vi "HelpBrowser.vi"() -> ()   [LabVIEW 2011]
uses:
  <vilib>/event_ctls.llb/eventvkey.ctl
panel:
  in  "Tab Control":T1(tab)
  in  "WebBrowser":refnum<k7>(container)
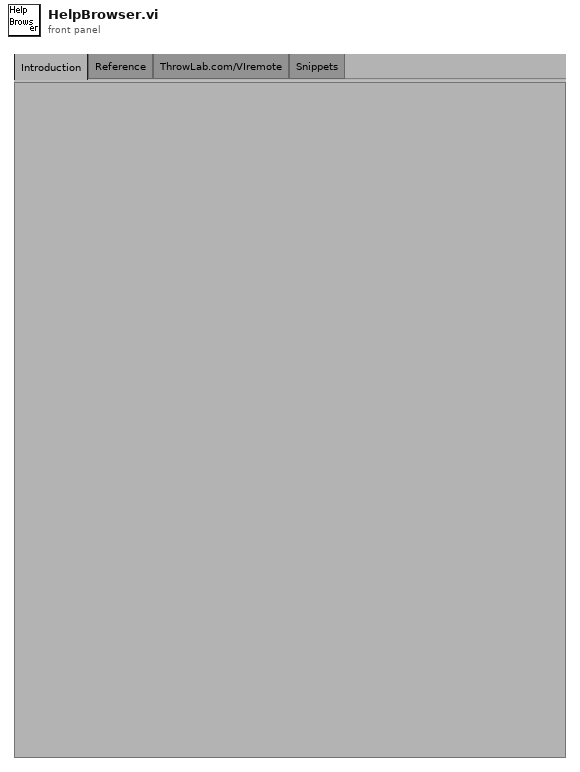
[diagram p1: front panel]
types:
  T1 = enum32{"Introduction", "Reference", "ThrowLab.com/VIremote", "Snippets"}
  T2 = typedef "eventvkey.ctl" = enum16{"ASCII", "Enter", "Return", "Shift", "Ctrl", "Alt", "Cmd", "Opt", "Caps", "NumLock", "Clear", "Break", "Up", "Down", "Left", "Right", "Insert", "Delete", "Home", "End", "PageUp", "PageDown", "Escape", "Help", "Pause", "ScrollLock", "F1", "F2", "F3", "F4", "F5", "F6", "F7", "F8", "F9", "F10", "F11", "F12", "F13", "F14", "F15", "F16", "F17", "F18", "F19", "F20", "F21", "F22", "F23", "F24", "Play", "VolumeUp", "VolumeDown", "Mute", "Two Byte Char"}
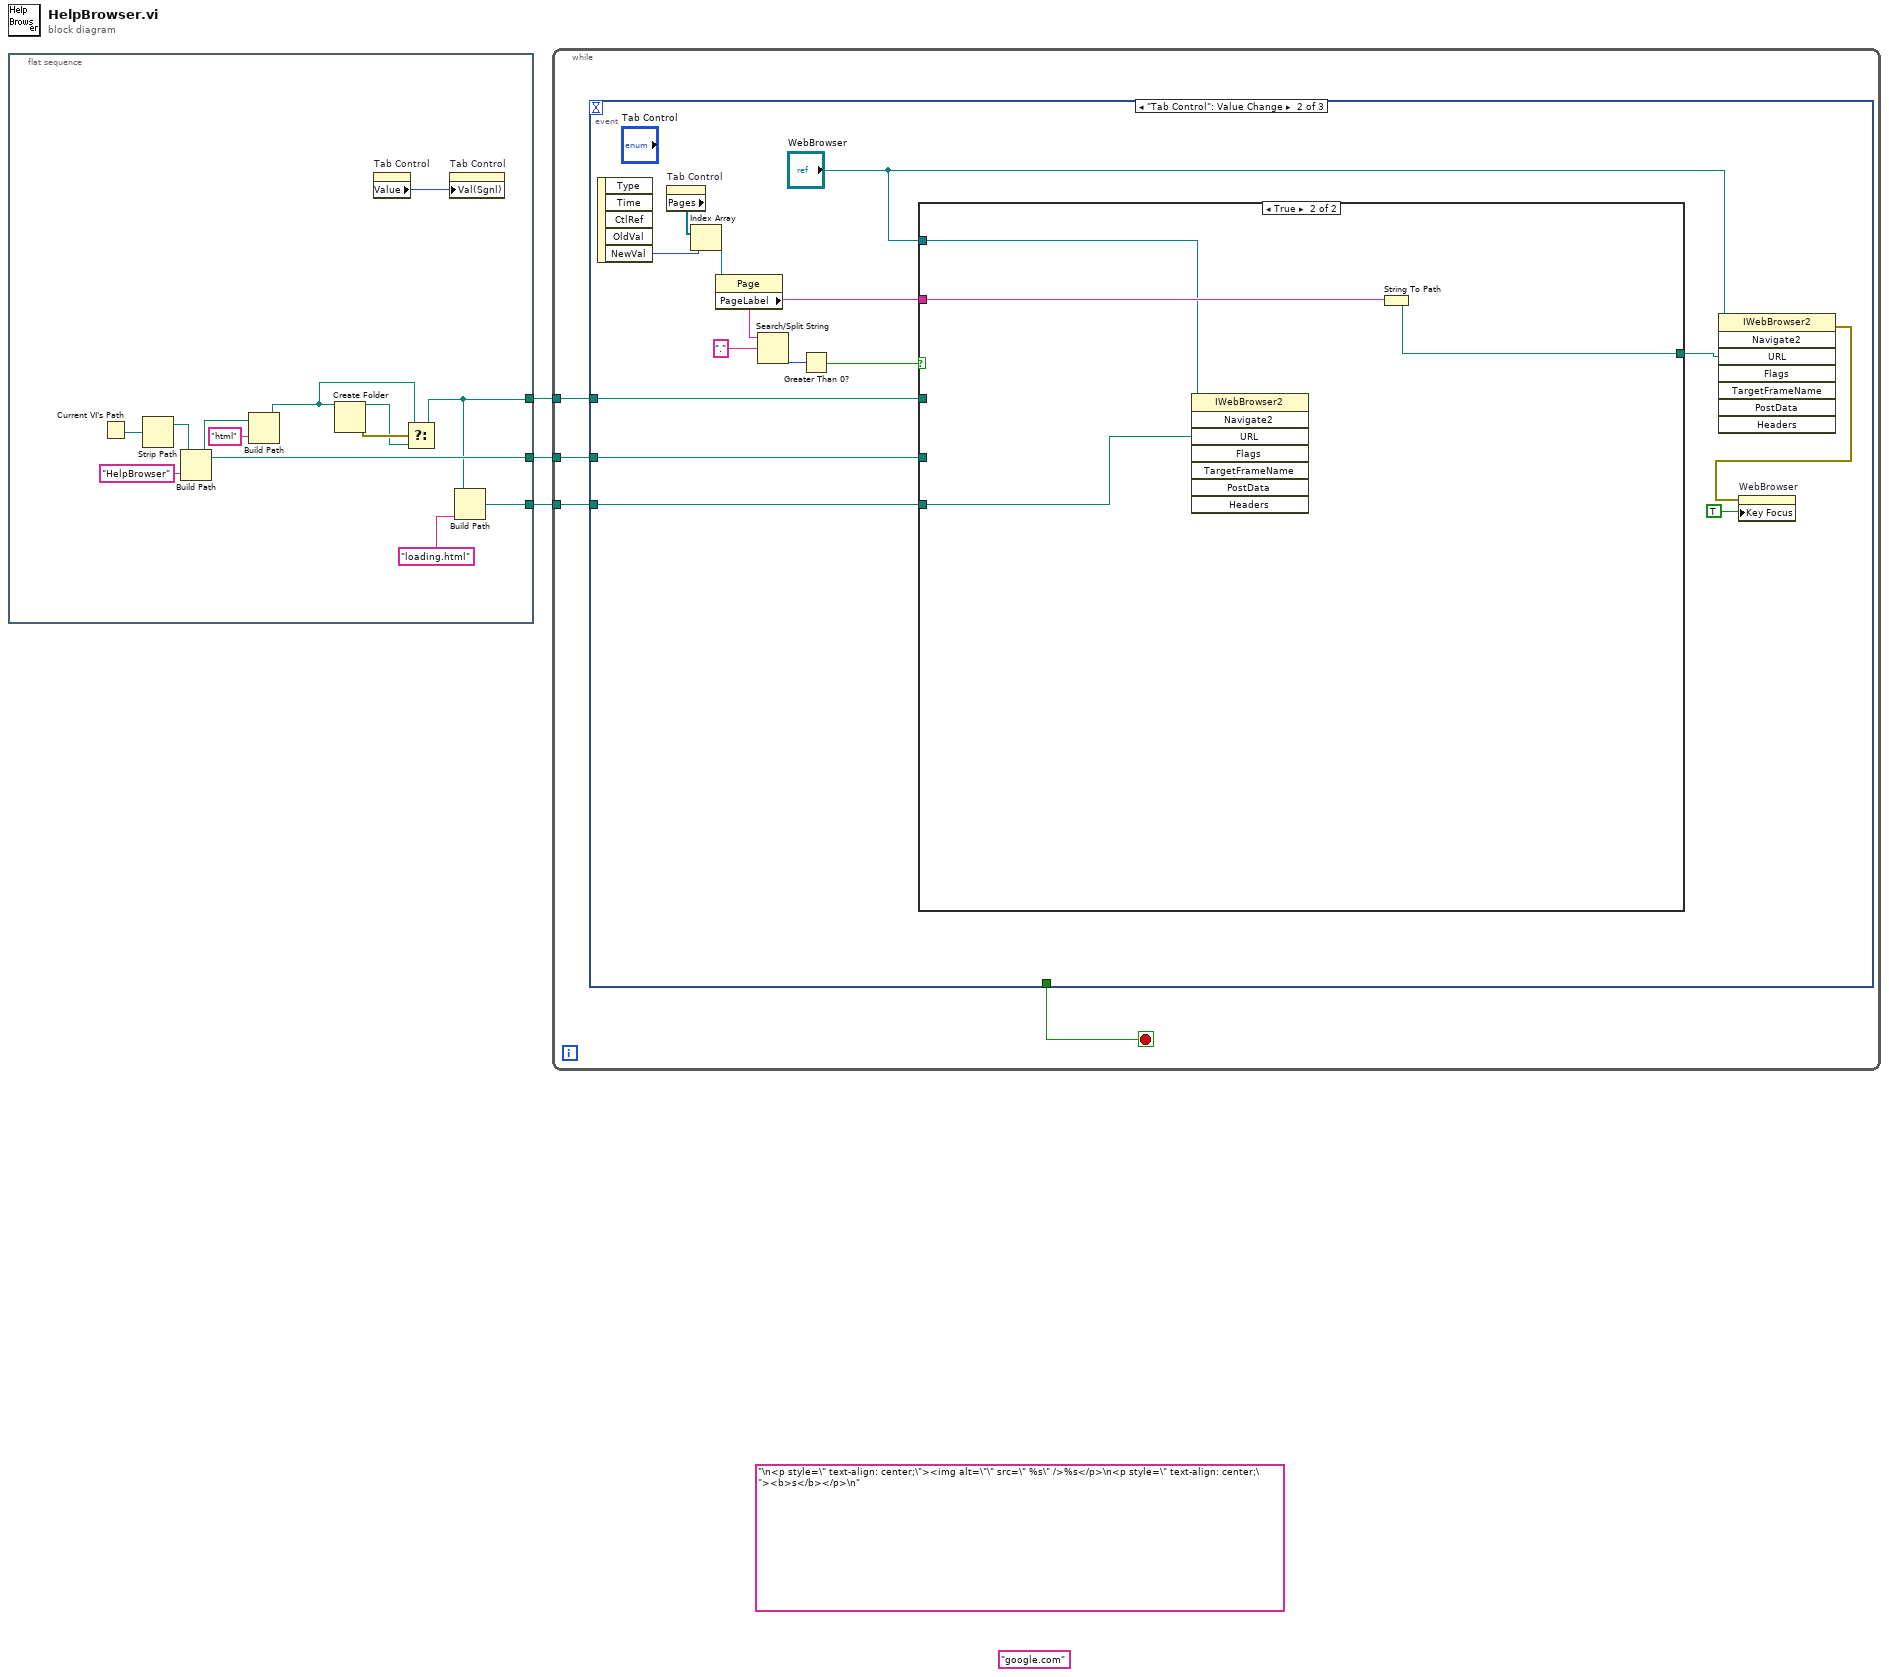
[diagram p0: block diagram]
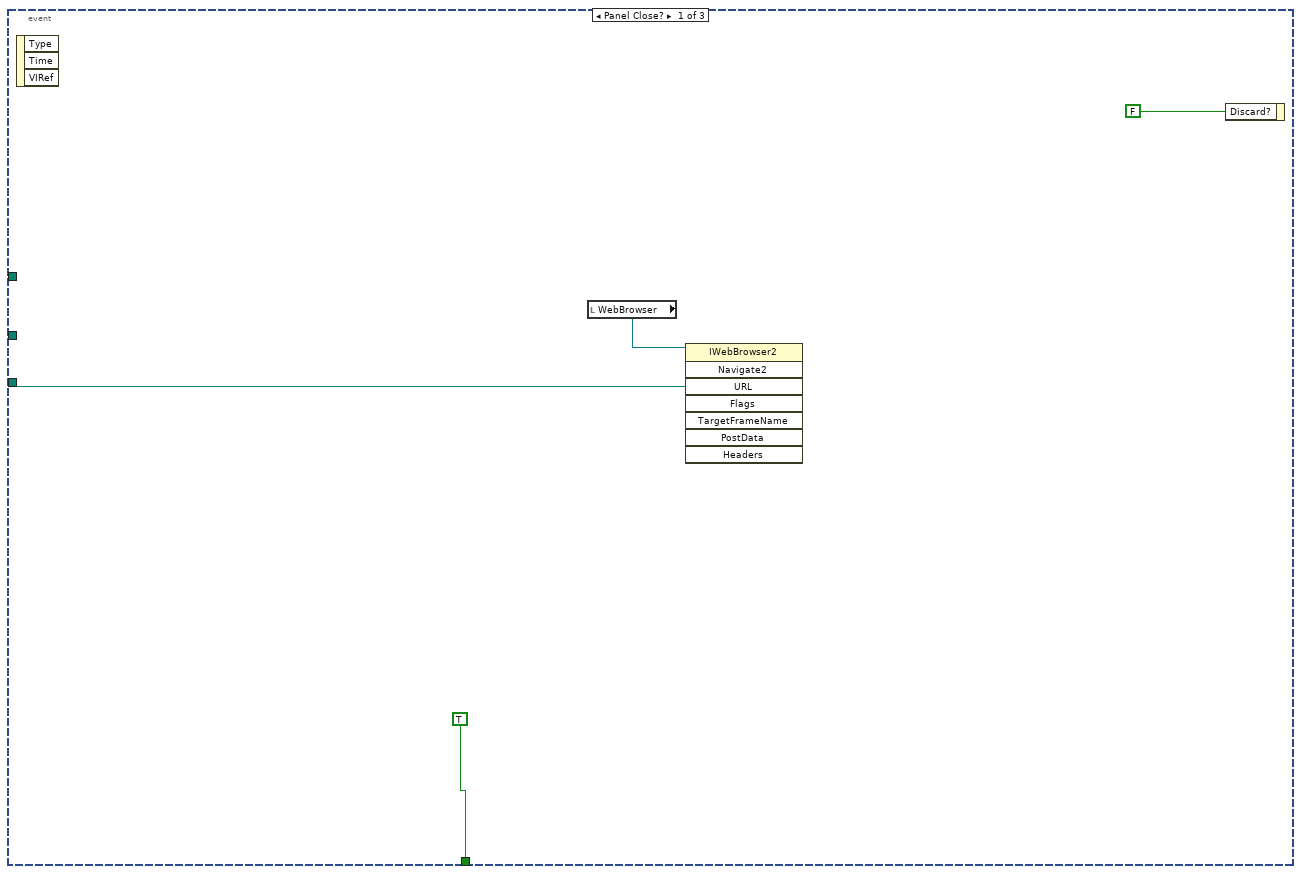
[diagram p2: hidden frame]
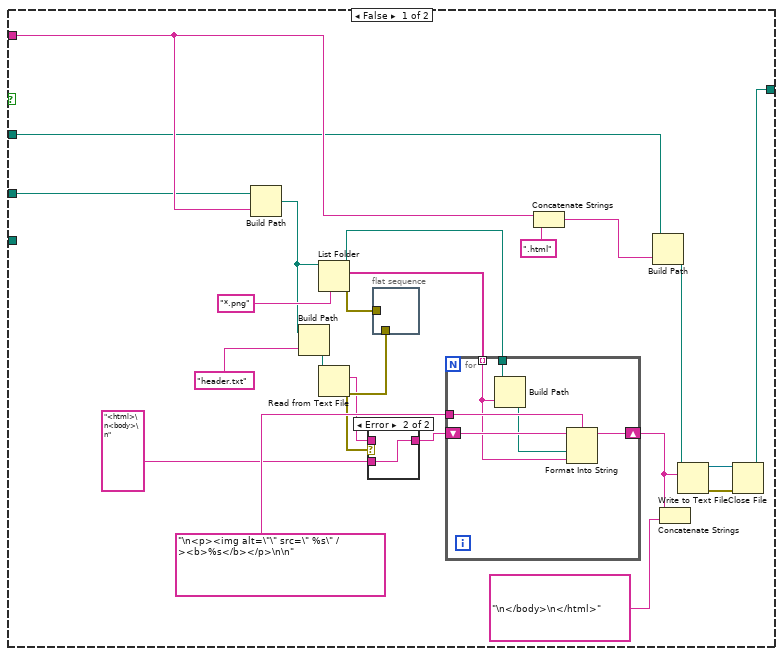
[diagram p3: hidden frame]
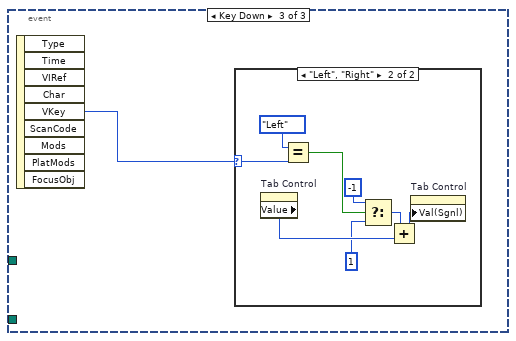
[diagram p5: hidden frame]
diagram:
  (unwired) "\n<p style=\" text-align: center;\"><img alt=\"\" src=\" %s\" />%s</p>\n<p style=\" text-align: center;\"><b>s</b></p>\n" ("name or relative path")
  (unwired) "google.com" ("URL")
  n1 = flat-sequence {
    tunnel: [w7] -> w3
    tunnel: [w5] -> w2
    tunnel: [w4] -> w1
    frame #0 {
      n2 = Current VI's Path() -> (path=w10:path)
      n3 = Strip Path(path=w10) -> (stripped path=w9:path)  [unwired: 1 out]
      n4 = Build Path(base path=w9, name or relative path="HelpBrowser") -> (appended path=w7:path)
      n5 = Build Path(base path=w7, name or relative path="html") -> (appended path=w14:path)
      n6 = Create Folder(path (use dialog)=w14) -> (created path=w12:path, error out=w13:errorcluster)  [unwired: 1 in, 2 out]
      n7 = property on="Tab Control" class="TabCtl (strict)"() -> ("Value"=w15:T1)  [unwired: 2 in, 2 out]
      n8 = Select(t=w14, s=w13, f=w12) -> (s? t:f=w5:path)
      n9 = property on="Tab Control" class="TabCtl (strict)"("Val(Sgnl)"=w15) -> ()  [unwired: 2 in, 2 out]
      n10 = Build Path(base path=w5, name or relative path="loading.html") -> (appended path=w4:path)
    }
  }
  n11 = while {
    tunnel: w2 -> [w18]
    tunnel: w3 -> [w17]
    tunnel: w1 -> [w16]
    stop <- w19 stop-if-true
    n12 = event shown="[1] \"Tab Control\": Value Change" {
      selector: _ -> [_ _ _]
      dyn-events: _ -> [_ _ _]
      timeout: _ -> [_ _ _]
      tunnel: [TRUE ("Discard?") _ _] -> w19
      tunnel: w18 -> [_ w27 _]
      tunnel: w17 -> [_ w26 _]
      tunnel: w16 -> [w21 w25 _]
      event Panel Close? {
        n13 = event-data() -> ()  [unwired: 4 out]
        n14 = local read "WebBrowser"() -> (w22:refnum<k7>)
        n15 = invoke class="IWebBrowser2" method="Navigate2"(reference=w22, "URL"=w21) -> ()  [unwired: 6 in, 8 out]
        n16 = event-data("Discard?"=FALSE) -> ()  [unwired: 1 in, 1 out]
      }
      event "Tab Control": Value Change {
        n17 = event-data() -> ("NewVal"=w37:T1)  [unwired: 5 out]
        n18 = property on="Tab Control" class="TabCtl (strict)"() -> ("Pages"=w36:refnum<vi>[])  [unwired: 2 in, 2 out]
        n19 = Index Array(array=w36, index=w37) -> (element=w35:refnum<vi>)
        n20 = property class="Page"(reference=w35) -> ("PageLabel"=w33:string)  [unwired: 1 in, 2 out]
        n21 = Search/Split String(string=w33, search string/char (-)=".") -> (offset of match=w31:i32)  [unwired: 3 out]
        n22 = Greater Than 0?(x=w31) -> (x > 0?=w30:bool)
        n23 = case shown="True" w30 {
          tunnel: [w57 w71] -> w34
          tunnel: w33 -> [w40 w72]
          tunnel: w26 -> [w39 _]
          tunnel: w27 -> [w38 _]
          tunnel: "WebBrowser" -> [_ w70]
          tunnel: w25 -> [_ w69]
          frame False {
            n24 = Build Path(base path=w39, name or relative path=w40) -> (appended path=w47:path)
            n25 = Build Path(base path=w47, name or relative path="header.txt" ("pattern")) -> (appended path=w48:path)
            n26 = List Folder(path=w47, pattern="*.png") -> (path out=w58:path, filenames=w53:string[], error out=w52:errorcluster)  [unwired: 1 in, 2 out]
            n27 = Read from Text File(file (use dialog)=w48) -> (text=w43:string, error out=w44:errorcluster)  [unwired: 1 in, 4 out]
            n28 = case shown="Error" w44 {
              tunnel: w43 -> [w61 _]
              tunnel: [w61 w62] -> w42
              tunnel: "<html>\n<body>\n" ("name or relative path") -> [_ w62]
              frame No Error {
              }
              frame Error {
              }
            }
            n29 = flat-sequence {
              tunnel: w52 -> [_]
              tunnel: w44 -> [_]
              frame #0 {
              }
            }
            n30 = for {
              tunnel: "\n<p><img alt=\"\" src=\" %s\" /><b>%s</b></p>\n\n" ("name or relative path") -> [w68]
              tunnel: w53 -> [w64] mode=indexing
              shift-right: [w67] -> w59
              shift-left: w42 -> [w66]
              tunnel: w58 -> [w65]
              n31 = Build Path(base path=w65, name or relative path=w64) -> (appended path=w63:path)
              n32 = Format Into String(format string=w68, initial string=w66, w63, w64) -> (resulting string=w67:string)  [unwired: 1 in, 1 out]
            }
            n33 = Concatenate Strings(w40, ".html" ("name or relative path")) -> (w50:string)
            n34 = Build Path(base path=w38, name or relative path=w50) -> (appended path=w54:path)
            n35 = Concatenate Strings(w59, "\n</body>\n</html>" ("name or relative path")) -> ()  [unwired: 1 out]
            n36 = Write to Text File(file (use dialog)=w54, text=w59) -> (refnum out=w56:refnum<file>, error out=w55:errorcluster)  [unwired: 1 in, 2 out]
            n37 = Close File(refnum=w56, error in=w55) -> (path=w57:path)  [unwired: 1 out]
          }
          frame True {
            n38 = invoke class="IWebBrowser2" method="Navigate2"(reference=w70, "URL"=w69) -> ()  [unwired: 6 in, 8 out]
            n39 = String To Path(string=w72) -> (path=w71:path)
          }
        }
        n40 = invoke class="IWebBrowser2" method="Navigate2"(reference="WebBrowser", "URL"=w34) -> (error out=w24:errorcluster)  [unwired: 6 in, 7 out]
        n41 = property on="WebBrowser" class="AXCont"(error in=w24, "Key Focus"=TRUE) -> ()  [unwired: 1 in, 2 out]
      }
      event Key Down {
        n42 = event-data() -> ("VKey"=w73:T2)  [unwired: 9 out]
        n43 = case shown="\"Left\", \"Right\"" w73 {
          selector: w73 -> [_ w80]
          frame "ASCII", Default {
          }
          frame "Left", "Right" {
            n44 = property on="Tab Control" class="TabCtl (strict)"() -> ("Value"=w76:T1)  [unwired: 2 in, 2 out]
            n45 = Equal?(x=eventvkey."Left" ("VKey"), y=w80) -> (x = y?=w79:bool)
            n46 = Select(t=-1, s=w79, f=1) -> (s? t:f=w78:i32)
            n47 = Add(x=w78, y=w76) -> (x+y=w77:u32)
            n48 = property on="Tab Control" class="TabCtl (strict)"("Val(Sgnl)"=w77) -> ()  [unwired: 2 in, 2 out]
          }
        }
      }
    }
  }
